vi "Read paper data.vi"(0 "Refnum in":T1, 11 "error in (no error)":errorcluster) -> (1 "Names":string[](array[string]), 2 "Costs":dbl[][](array[numeric]), 3 "Days":bool[][](array[boolean]), 4 "Refnum out":T1, 15 "error out":errorcluster)   [LabVIEW 2015]
uses:
  <vilib>/Utility/config.llb/Config Data RefNum.ctl
  <vilib>/Utility/config.llb/Read Key (Path).vi
  <vilib>/Utility/file.llb/Read Delimited Spreadsheet (string).vi
  <vilib>/Utility/file.llb/Read Delimited Spreadsheet (DBL).vi
  <vilib>/Utility/config.llb/NI_LVConfig.lvlib
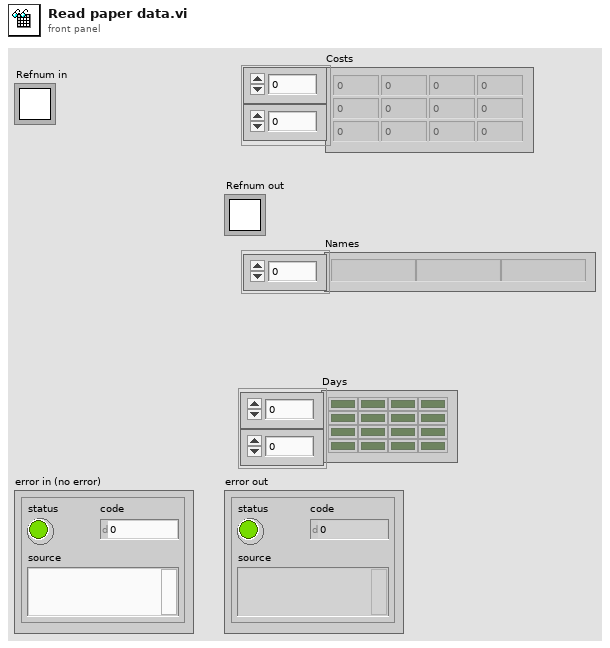
[diagram p1: front panel]
types:
  T1 = typedef "NI_LVConfig.lvlib/Config Data RefNum.ctl" = refnum<k1>
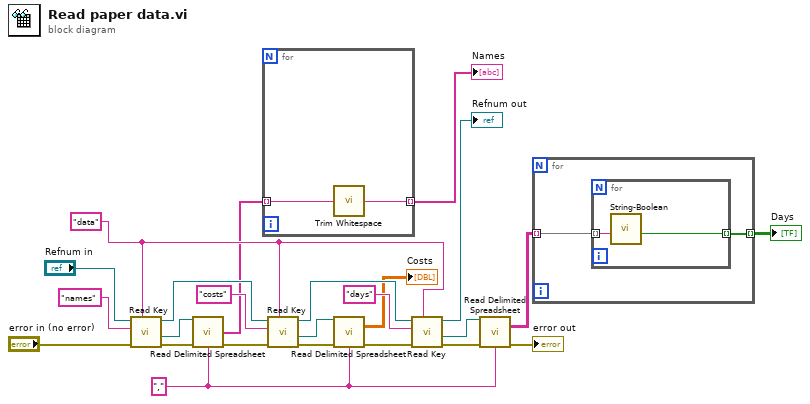
[diagram p0: block diagram]
diagram:
  w3 = "," ("delimiter (\\t)")
  w15 = "data" ("section")
  n1 = call-poly <vilib>:"Read Key.vi"("section"=w15, "error in (no error)"="error in (no error)", "key"="names", "refnum"="Refnum in") -> ("error out"=w19:errorcluster, "value"=w8:path, "refnum out"=w18:T1)  [unwired: 4 in, 1 out]
  n2 = call-poly <vilib>:"Read Delimited Spreadsheet.vi"("file path (dialog if empty)"=w8, "error in (no error)"=w19, "delimiter (\\t)"=w3) -> ("first row"=w2:string[], "error out"=w11:errorcluster)  [unwired: 7 in, 4 out]
  n3 = for {
    tunnel: w2 -> [w26] mode=indexing
    tunnel: [w25] -> w1 mode=indexing
    n4 = call <vilib>:"Trim Whitespace.vi"("string"=w26) -> ("trimmed string"=w25:string)  [unwired: 1 in]
  }
  "Names" <- w1
  n5 = call-poly <vilib>:"Read Key.vi"("section"=w15, "error in (no error)"=w11, "key"="costs", "refnum"=w18) -> ("error out"=w17:errorcluster, "value"=w7:path, "refnum out"=w16:T1)  [unwired: 4 in, 1 out]
  n6 = call-poly <vilib>:"Read Delimited Spreadsheet.vi"("file path (dialog if empty)"=w7, "error in (no error)"=w17, "delimiter (\\t)"=w3) -> ("all rows"=→"Costs":dbl[][], "error out"=w10:errorcluster)  [unwired: 7 in, 4 out]
  n7 = call-poly <vilib>:"Read Key.vi"("section"=w15, "error in (no error)"=w10, "key"="days", "refnum"=w16) -> ("error out"=w9:errorcluster, "value"=w6:path, "refnum out"=→"Refnum out":T1)  [unwired: 4 in, 1 out]
  n8 = call-poly <vilib>:"Read Delimited Spreadsheet.vi"("file path (dialog if empty)"=w6, "error in (no error)"=w9, "delimiter (\\t)"=w3) -> ("all rows"=w4:string[][], "error out"=→"error out":errorcluster)  [unwired: 7 in, 4 out]
  n9 = for {
    tunnel: w4 -> [w28] mode=indexing
    tunnel: [w27] -> w20 mode=indexing
    n10 = for {
      tunnel: w28 -> [w30] mode=indexing
      tunnel: [w29] -> w27 mode=indexing
      n11 = call "String-Boolean.vi"("String in"=w30) -> ("Boolean out"=w29:bool)  [unwired: 9 in, 1 out]
    }
  }
  "Days" <- w20
